vi "Add_Update_Values.vi"(0 "Filename":path, 1 "Value  Constant?":bool, 2 "Edit Raw data files?":bool, 3 "Filetype":string, 5 "New Chs In":string[](array[string])=[""], 7 "Edit Raw Data Header Info":bool, 9 "New Values In":string[][](array[string]), 11 "Selected Rows":i32[](array[numeric]), 12 "Edit all Rows?":bool, 13 "Raw DF in Orig Pos?":bool, 14 "Job Directory":path=path "/G4_2_HD/Users/paulhayden/Documents/Projects/Hong Roughness/XW data/XW_Corr.tpt") -> ()   [LabVIEW 2021]
panel:
  in  "Warn If files not found?":bool=TRUE
  out "Checking Raw data files":i32
  in  "stop":bool
  out "Currently editing":string
  out "Folder Containing Raw data Files":path
  out "size(s)":i32
  out "Files Processed":i32(slide) scale=0.0..522.0
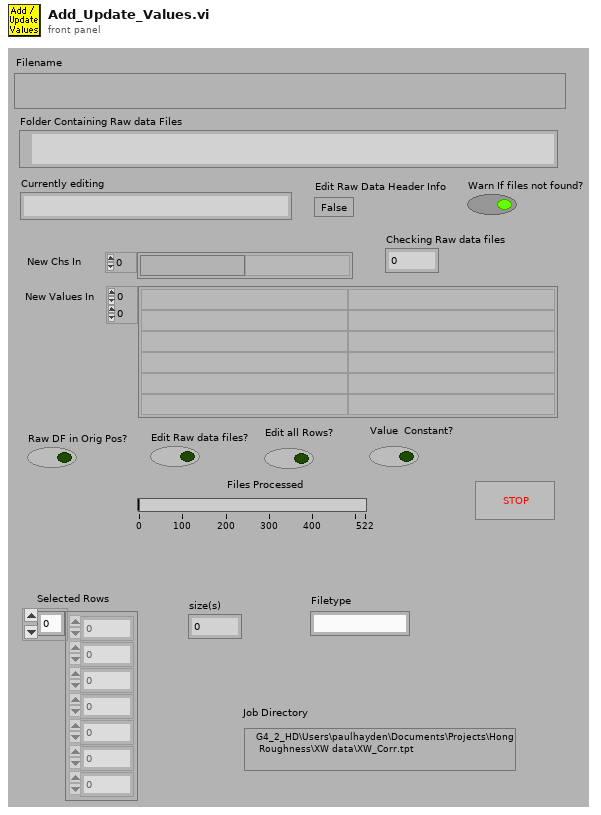
[diagram p1: front panel]
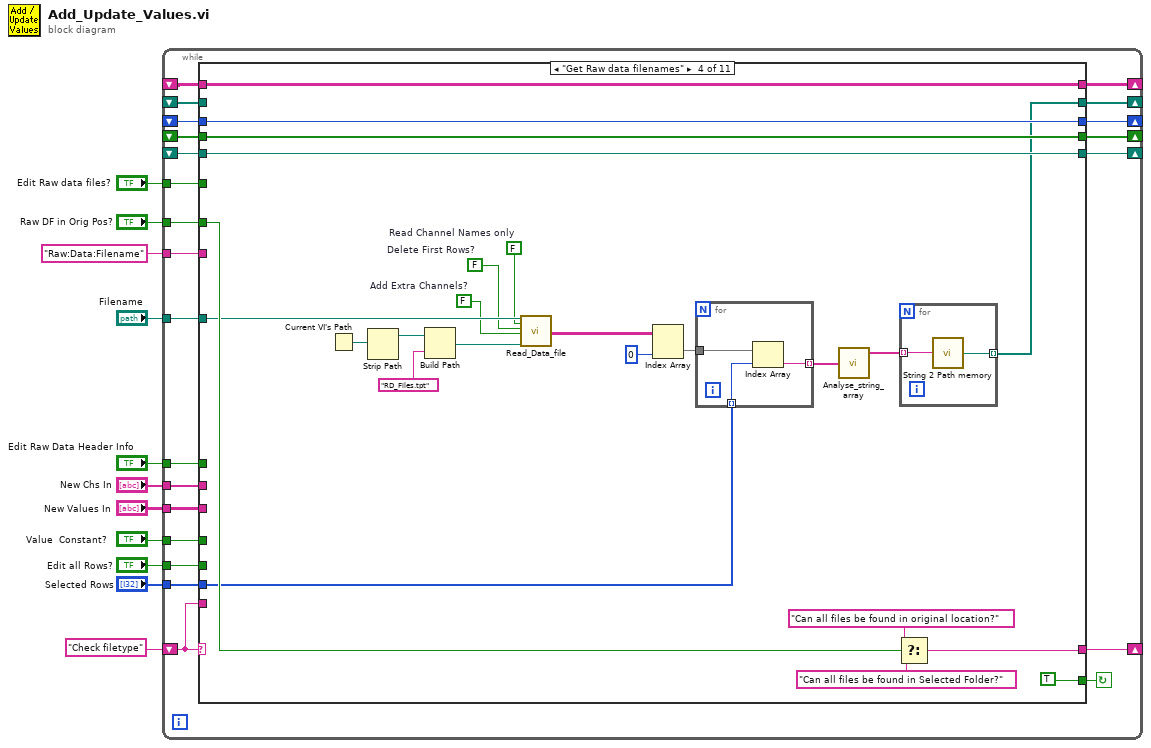
[diagram p0: block diagram]
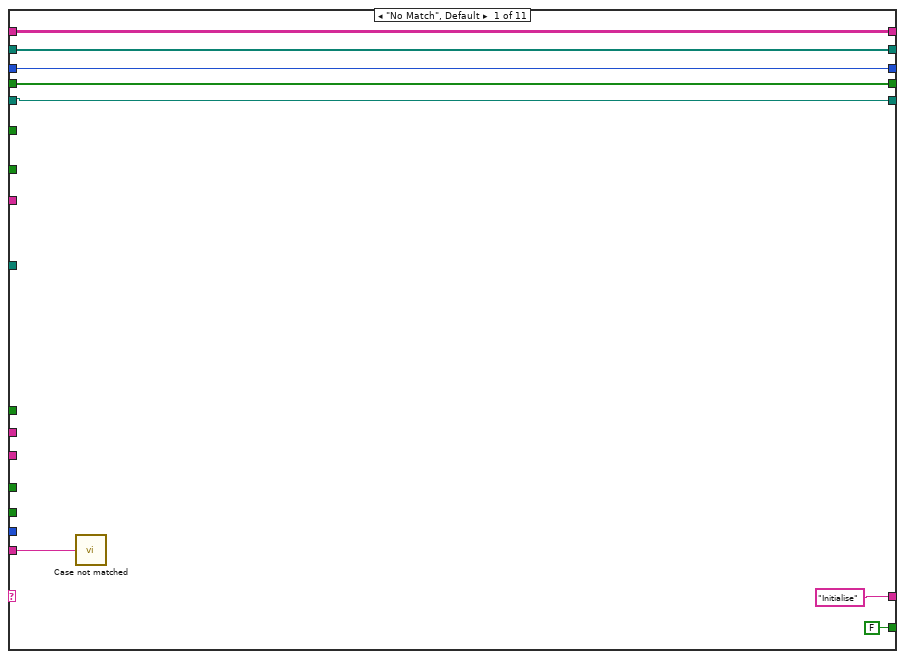
[diagram p2: hidden frame]
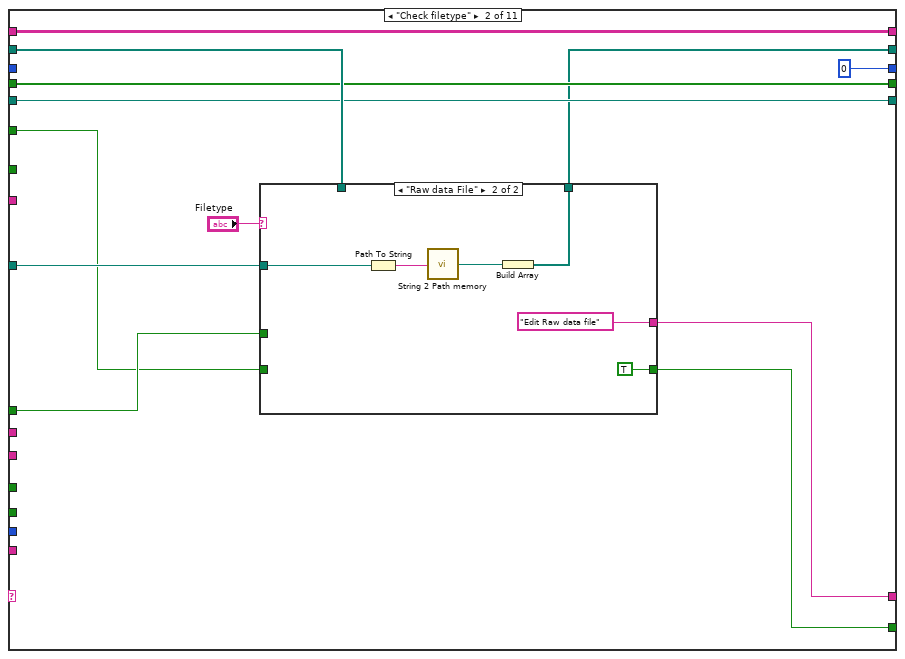
[diagram p3: hidden frame]
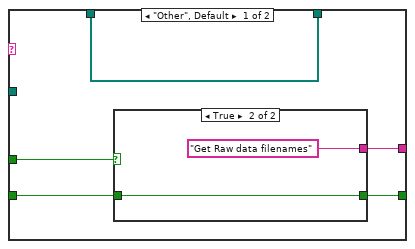
[diagram p4: hidden frame]
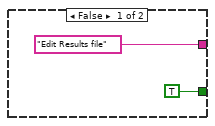
[diagram p5: hidden frame]
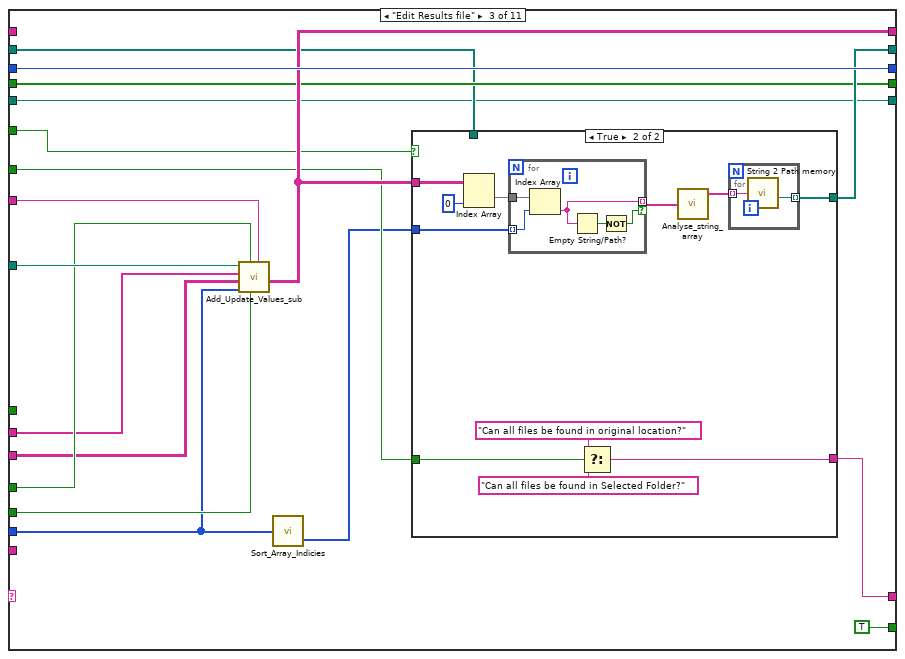
[diagram p6: hidden frame]
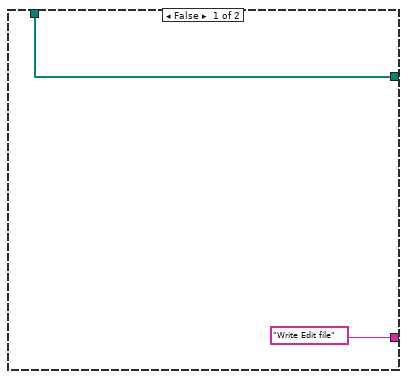
[diagram p7: hidden frame]
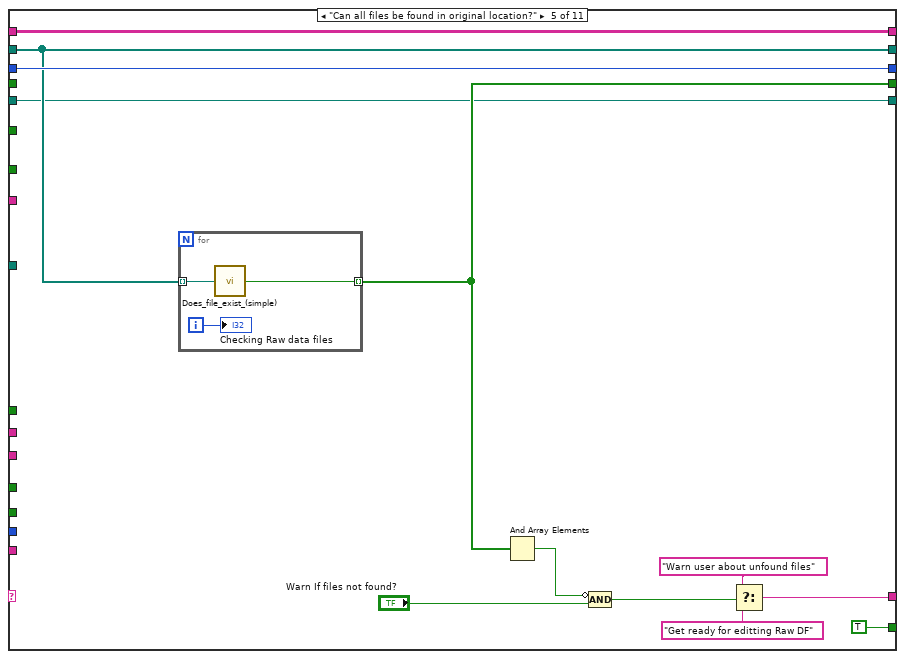
[diagram p8: hidden frame]
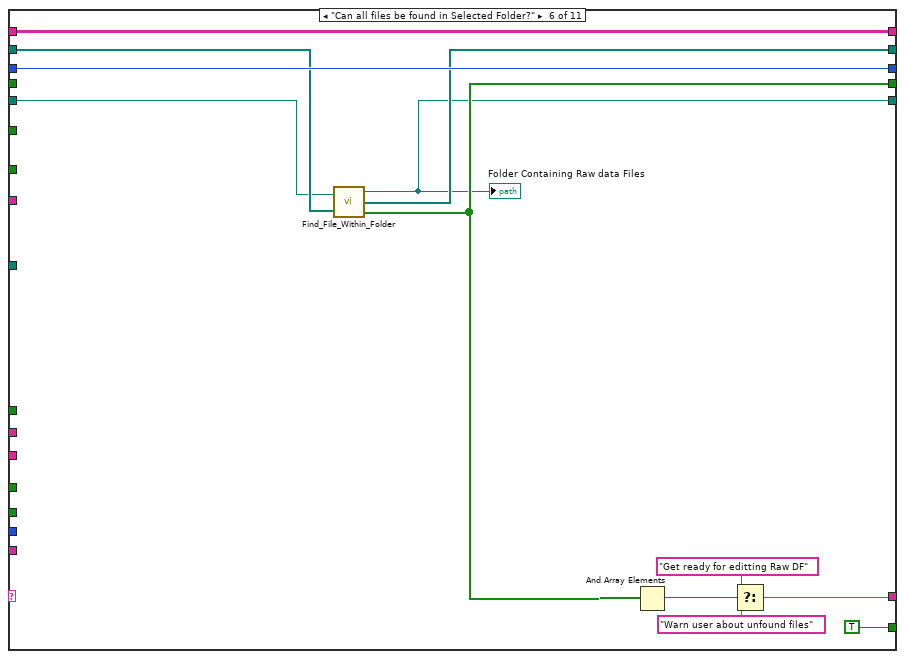
[diagram p9: hidden frame]
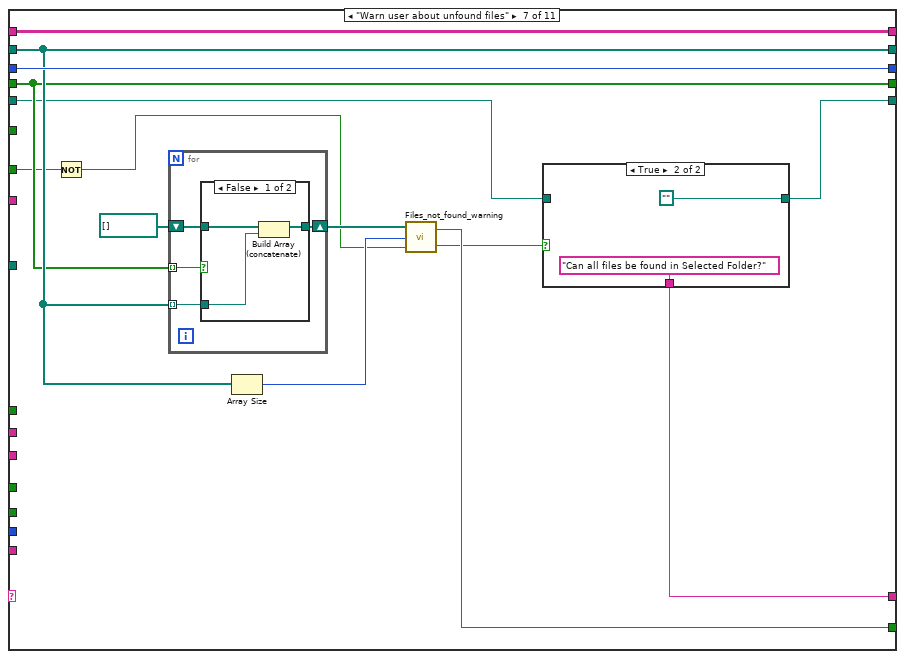
[diagram p10: hidden frame]
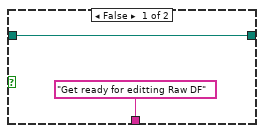
[diagram p11: hidden frame]
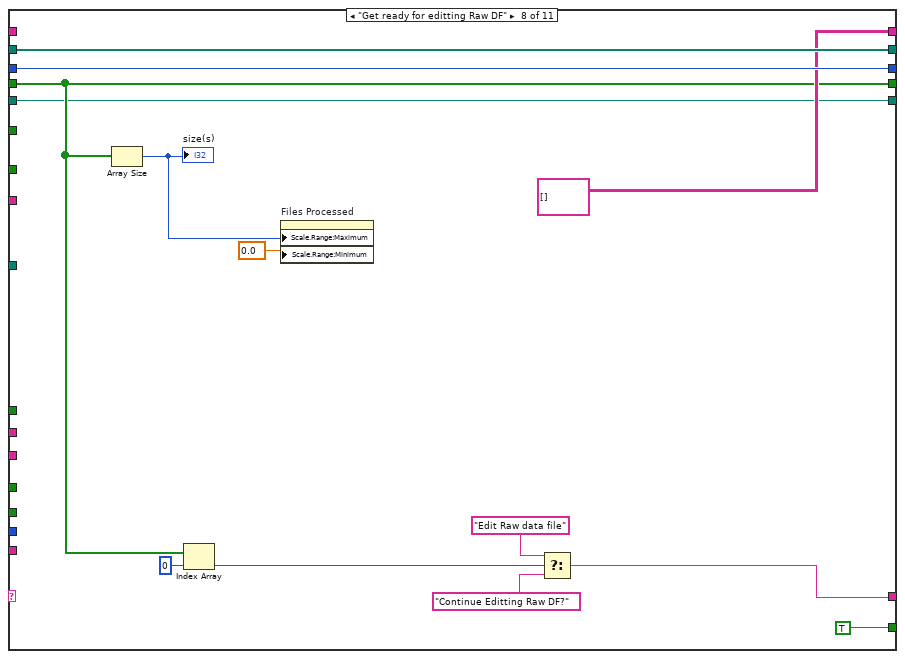
[diagram p13: hidden frame]
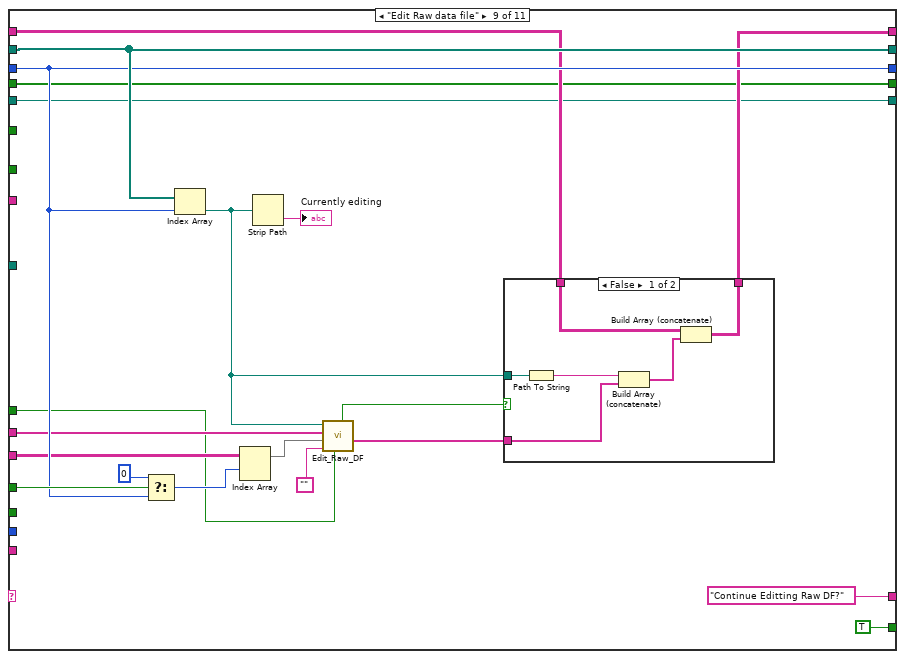
[diagram p14: hidden frame]
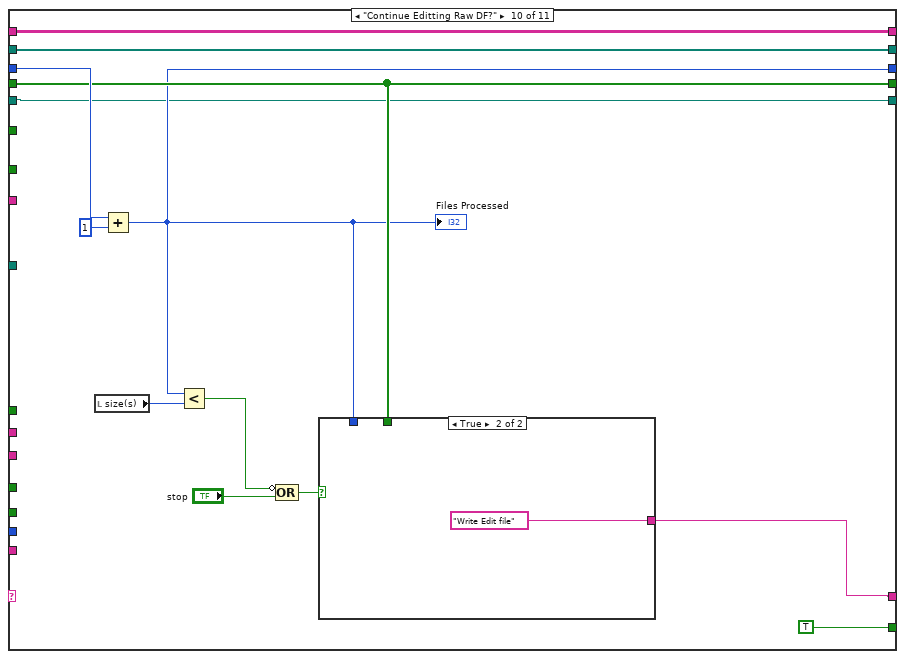
[diagram p16: hidden frame]
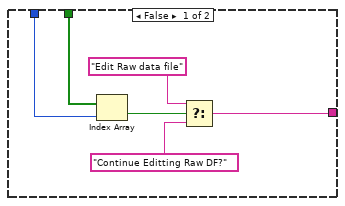
[diagram p17: hidden frame]
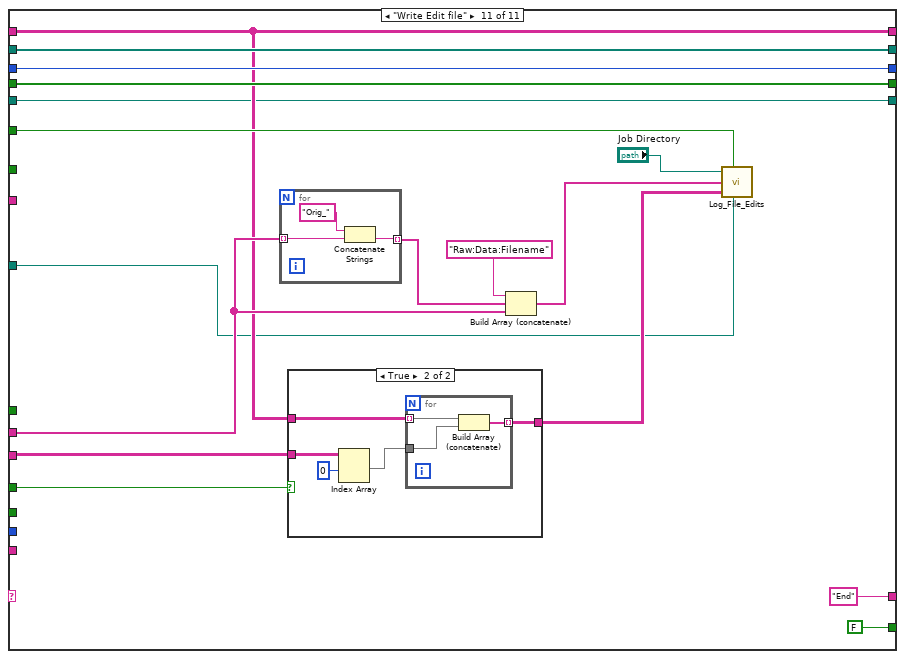
[diagram p18: hidden frame]
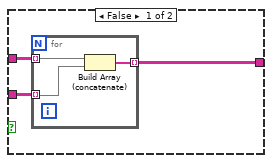
[diagram p19: hidden frame]
diagram:
  n1 = while {
    shift-left: "Check filetype" -> [w32]
    shift-right: [w33] -> _
    shift-right: [w30] -> _
    shift-left: _ -> [w29]
    tunnel: "Filename" -> [w31]
    shift-right: [w28] -> _
    shift-left: _ -> [w27]
    tunnel: "Value  Constant?" -> [w26]
    tunnel: "Edit Raw Data Header Info" -> [w25]
    shift-right: [w24] -> _
    shift-left: _ -> [w23]
    tunnel: "New Chs In" -> [w22]
    tunnel: "New Values In" -> [w21]
    tunnel: "Edit all Rows?" -> [w20]
    shift-right: [w19] -> _
    shift-left: _ -> [w18]
    tunnel: "Edit Raw data files?" -> [w17]
    tunnel: "Raw DF in Orig Pos?" -> [w16]
    shift-right: [w14] -> _
    shift-left: _ -> [w15]
    tunnel: "Selected Rows" -> [w13]
    tunnel: "Raw:Data:Filename" -> [w12]
    stop <- w34 continue-if-true
    n2 = case shown="\"Get Raw data filenames\"" w32 {
      tunnel: [FALSE w45 TRUE TRUE TRUE TRUE w171 TRUE TRUE TRUE FALSE] -> w34
      tunnel: ["Initialise" w52 w76 w128 w143 w154 w167 w194 "Continue Editting Raw DF?" ("t") w234 "End" ("t")] -> w33
      tunnel: w32 -> [w35 _ _ _ _ _ _ _ _ _ _]
      tunnel: w31 -> [_ w50 w85 w117 _ _ _ _ _ _ w252]
      tunnel: [w39 w43 w79 w111 w146 w160 w173 w200 w219 w240 w265] -> w30
      tunnel: w29 -> [w39 w53 w75 _ w146 w159 w173 w200 w219 w240 w265]
      tunnel: [w40 0 w87 w131 w148 w163 w177 w202 w218 w235 w263] -> w28
      tunnel: w27 -> [w40 _ w87 w131 w148 w163 w177 w202 w218 w239 w263]
      tunnel: w26 -> [_ _ w84 _ _ _ _ _ w222 _ w253]
      tunnel: w25 -> [_ w46 _ _ _ _ _ _ w204 _ _]
      tunnel: [w38 w49 w80 w123 w145 w161 w175 string[][] [] ("Edit Info") w209 w241 w256] -> w24
      tunnel: w23 -> [w38 w49 _ w123 w145 w161 w175 _ w210 w241 w256]
      tunnel: w22 -> [_ _ w83 _ _ _ _ _ w216 _ w258]
      tunnel: w21 -> [_ _ w82 _ _ _ _ _ w215 _ w255]
      tunnel: w20 -> [_ _ w81 _ _ _ _ _ _ _ _]
      tunnel: [w37 w48 w78 w129 w144 w155 w172 w198 w208 w236 w264] -> w19
      tunnel: w18 -> [w37 w48 w78 w129 _ _ w172 w198 w208 w236 w264]
      tunnel: w17 -> [_ w44 w77 _ _ _ _ _ _ _ w260]
      tunnel: w16 -> [_ _ w74 w127 _ _ w170 _ _ _ _]
      tunnel: w15 -> [w36 w47 w73 w126 w142 w153 w164 w190 w205 w230 w250]
      tunnel: [w36 w47 w73 w126 w142 w152 w165 w190 w205 w230 w250] -> w14
      tunnel: w13 -> [_ _ w71 w122 _ _ _ _ _ _ _]
      tunnel: w12 -> [_ _ w72 _ _ _ _ _ _ _ _]
      frame "No Match", Default {
        n3 = call "Case not matched.vi"("Case Name not Matched"=w35) -> ()
      }
      frame "Check filetype" {
        n4 = case shown="\"Raw data File\"" "Filetype" {
          tunnel: w50 -> [_ w67]
          tunnel: w53 -> [w55 _]
          tunnel: [w58 "Edit Raw data file"] -> w52
          tunnel: w46 -> [w59 _]
          tunnel: [w57 TRUE ("Edit Raw data files?")] -> w45
          tunnel: w44 -> [w56 _]
          tunnel: [w55 w64] -> w43
          frame "Other", Default {
            n5 = case shown="True" w59 {
              tunnel: ["Edit Results file" "Get Raw data filenames"] -> w58
              tunnel: [TRUE ("Edit Raw data files?") w62] -> w57
              tunnel: w56 -> [_ w62]
              frame False {
              }
              frame True {
              }
            }
          }
          frame "Raw data File" {
            n6 = Path To String(path=w67) -> (string=w66:string)
            n7 = call "String 2 Path memory.vi"("Input String"=w66) -> ("path"=w65:path)  [unwired: 1 in]
            n8 = Build Array(w65) -> (w64:path[])
          }
        }
      }
      frame "Edit Results file" {
        n9 = call "Add_Update_Values_sub.vi"("Raw data Filename column name"=w72, "Edit all Rows?"=w81, "Value  Constant?"=w84, "Selected Rows"=w71, "New Values In"=w82, "New Chs In"=w83, "Filename"=w85) -> ("Edit Info"=w80:string[][])  [unwired: 4 out]
        n10 = call "Sort_Array_Indicies.vi"("unsorted array"=w71) -> ("Sort Index"=w70:i32[])  [unwired: 1 out]
        n11 = case shown="True" w77 {
          tunnel: w80 -> [_ w100]
          tunnel: [w88 w90] -> w79
          tunnel: w74 -> [_ w98]
          tunnel: ["Write Edit file" w95] -> w76
          tunnel: w75 -> [w88 _]
          tunnel: w70 -> [_ w93]
          frame False {
          }
          frame True {
            n12 = Index Array(array=w100, index (col)=0 ("disabled index (col)")) -> (element=w94:string[])  [unwired: 1 in]
            n13 = for {
              tunnel: [w103] -> w92 mode=indexing if=w104
              tunnel: w94 -> [w107]
              tunnel: w93 -> [w106] mode=indexing
              n14 = Index Array(array=w107, index=w106) -> (element=w103:string)
              n15 = Empty String/Path?(string/path=w103) -> (empty?=w105:bool)
              n16 = Not(x=w105) -> (.not. x?=w104:bool)
            }
            n17 = Select(t="Can all files be found in original location?", s=w98, f="Can all files be found in Selected Folder?") -> (s? t:f=w95:string)
            n18 = call "Analyse_string_array.vi"("String array"=w92) -> ("Unique strings"=w91:string[])  [unwired: 1 in, 1 out]
            n19 = for {
              tunnel: [w102] -> w90 mode=indexing
              tunnel: w91 -> [w101] mode=indexing
              n20 = call "String 2 Path memory.vi"("Input String"=w101) -> ("path"=w102:path)  [unwired: 1 in]
            }
          }
        }
      }
      frame "Get Raw data filenames" {
        w110 = FALSE  # Delete First Rows?
        w114 = FALSE  # Add Extra Channels?
        w115 = FALSE  # Read Channel Names only
        n21 = Current VI's Path() -> (path=w120:path)
        n22 = Strip Path(path=w120) -> (stripped path=w119:path)  [unwired: 1 out]
        n23 = Build Path(base path=w119, name or relative path="RD_Files.tpt") -> (appended path=w116:path)
        n24 = call "Read_Data_file.vi"("Results file"=w117, "Read Channel Names only"=w115, "Delete First Rows?"=w110, "Add Extra Channels?"=w114, "Template File"=w116) -> ("Channel Values Out"=w113:string[][])  [unwired: 2 in, 12 out]
        n25 = Index Array(array=w113, index (col)=0 ("index (row)")) -> (element=w121:string[])  [unwired: 1 in]
        n26 = for {
          tunnel: w122 -> [w136] mode=indexing
          tunnel: w121 -> [w135]
          tunnel: [w134] -> w109 mode=indexing
          n27 = Index Array(array=w135, index=w136) -> (element=w134:string)
        }
        n28 = call "Analyse_string_array.vi"("String array"=w109) -> ("Unique strings"=w108:string[])  [unwired: 1 in, 1 out]
        n29 = Select(t="Can all files be found in original location?", s=w127, f="Can all files be found in Selected Folder?") -> (s? t:f=w128:string)
        n30 = for {
          tunnel: [w133] -> w111 mode=indexing
          tunnel: w108 -> [w132] mode=indexing
          n31 = call "String 2 Path memory.vi"("Input String"=w132) -> ("path"=w133:path)  [unwired: 1 in]
        }
      }
      frame "Can all files be found in original location?" {
        n32 = for {
          tunnel: w146 -> [w151] mode=indexing
          tunnel: [w150] -> w144 mode=indexing
          i -> [w149]
          n33 = call "Does_file_exist_(simple).vi"("Pathname"=w151) -> ("exists?"=w150:bool)
          "Checking Raw data files" <- w149
        }
        n34 = And Array Elements(Boolean array=w144) -> (logical AND=w141:bool)
        n35 = Compound Arithmetic op=AND(invert w141, "Warn If files not found?") -> (w139:bool)
        n36 = Select(t="Warn user about unfound files", s=w139, f="Get ready for editting Raw DF" ("t")) -> (s? t:f=w143:string)
      }
      frame "Can all files be found in Selected Folder?" {
        n37 = call "Find_File_Within_Folder.vi"("Folder to Search"=w153, "Files to find"=w159) -> ("Folder to Search Out"=w152:path, "New File Paths"=w160:path[], "Files Found?"=w155:bool[])
        "Folder Containing Raw data Files" <- w152
        n38 = And Array Elements(Boolean array=w155) -> (logical AND=w158:bool)
        n39 = Select(t="Get ready for editting Raw DF", s=w158, f="Warn user about unfound files") -> (s? t:f=w154:string)
      }
      frame "Warn user about unfound files" {
        n40 = Not(x=w170) -> (.not. x?=w169:bool)
        n41 = for {
          tunnel: w173 -> [w182] mode=indexing
          shift-right: [w185] -> w174
          shift-left: path[] [] -> [w184]
          tunnel: w172 -> [w183] mode=indexing
          n42 = case shown="False" w183 {
            tunnel: w184 -> [w188 w189]
            tunnel: [w186 w189] -> w185
            tunnel: w182 -> [w187 _]
            frame False {
              n43 = Build Array (concatenate)(w188, w187) -> (w186:path[])
            }
            frame True {
            }
          }
        }
        n44 = Array Size(array=w173) -> (size(s)=w176:i32)
        n45 = call "Files_not_found_warning.vi"("Use Selected Folder?"=w169, "Total number of data files"=w176, "Unfound Files"=w174) -> ("Edit Selected Folder Out"=w168:bool, "Edit Files?"=w171:bool)
        n46 = case shown="True" w168 {
          tunnel: ["Get ready for editting Raw DF" ("t") "Can all files be found in Selected Folder?" ("t")] -> w167
          tunnel: [w178 path ""] -> w165
          tunnel: w164 -> [w178 _]
          frame False {
          }
          frame True {
          }
        }
      }
      frame "Get ready for editting Raw DF" {
        n47 = Array Size(array=w198) -> (size(s)=w191:i32)
        "size(s)" <- w191
        n48 = Index Array(array=w198, index=0) -> (element=w196:bool)
        n49 = property on="Files Processed" class="Slide (strict)"("Scale.Range:Maximum"=w191, "Scale.Range:Minimum"=0.0 ("Scale.Range:Maximum")) -> ()  [unwired: 2 in, 2 out]
        n50 = Select(t="Edit Raw data file", s=w196, f="Continue Editting Raw DF?") -> (s? t:f=w194:string)
      }
      frame "Edit Raw data file" {
        n51 = Select(t=0, s=w222, f=w218) -> (s? t:f=w220:i32)
        n52 = Index Array(array=w219, index=w218) -> (element=w207:path)
        n53 = Index Array(array=w215, index (row)=w220) -> (element=w214:string[])  [unwired: 1 in]
        n54 = Strip Path(path=w207) -> (name=→"Currently editing":string)  [unwired: 1 out]
        n55 = call "Edit_Raw_DF.vi"("Edit Raw Data Header Info"=w204, "New Analysis Info Cluster Setup"="", "New Values In"=w214, "New Chs In"=w216, "Data filename"=w207) -> ("Original values"=w212:string[], "File Not Changed?"=w211:bool)  [unwired: 1 in, 2 out]
        n56 = case shown="False" w211 {
          tunnel: w207 -> [w228 _]
          tunnel: w212 -> [w226 _]
          tunnel: w210 -> [w224 w229]
          tunnel: [w223 w229] -> w209
          frame False {
            n57 = Path To String(path=w228) -> (string=w227:string)
            n58 = Build Array (concatenate)(w227, w226) -> (w225:string[])
            n59 = Build Array (concatenate)(w224, w225) -> (w223:string[][])
          }
          frame True {
          }
        }
      }
      frame "Continue Editting Raw DF?" {
        n60 = local read "size(s)"() -> (w237:i32)
        n61 = Add(x=w239, y=1) -> (x+y=w235:i32)
        "Files Processed" <- w235
        n62 = Less?(x=w235, y=w237) -> (x < y?=w232:bool)
        n63 = Compound Arithmetic op=OR(invert w232, "stop") -> (w231:bool)
        n64 = case shown="True" w231 {
          tunnel: w236 -> [w247 _]
          tunnel: w235 -> [w246 _]
          tunnel: [w244 "Write Edit file" ("t")] -> w234
          frame False {
            n65 = Index Array(array=w247, index=w246) -> (element=w248:bool)
            n66 = Select(t="Edit Raw data file", s=w248, f="Continue Editting Raw DF?") -> (s? t:f=w244:string)
          }
          frame True {
          }
        }
      }
      frame "Write Edit file" {
        n67 = for {
          tunnel: w258 -> [w283] mode=indexing
          tunnel: [w281] -> w259 mode=indexing
          n68 = Concatenate Strings("Orig_" ("string"), w283) -> (w281:string)
        }
        n69 = case shown="True" w253 {
          tunnel: w256 -> [w269 w277]
          tunnel: w255 -> [w268 w275]
          tunnel: [w267 w276] -> w254
          frame False {
            n70 = for {
              tunnel: w269 -> [w272] mode=indexing
              tunnel: w268 -> [w271] mode=indexing
              tunnel: [w270] -> w267 mode=indexing
              n71 = Build Array (concatenate)(w272, w271) -> (w270:string[])
            }
          }
          frame True {
            n72 = Index Array(array=w275, index (row)=0) -> (element=w273:string[])  [unwired: 1 in]
            n73 = for {
              tunnel: w277 -> [w280] mode=indexing
              tunnel: [w279] -> w276 mode=indexing
              tunnel: w273 -> [w278]
              n74 = Build Array (concatenate)(w280, w278) -> (w279:string[])
            }
          }
        }
        n75 = Build Array (concatenate)("Raw:Data:Filename", w259, w258) -> (w257:string[])
        n76 = call "Log_File_Edits.vi"("Job Directory"="Job Directory", "File Editted?"=w260, "Channels to Edit"=w257, "Data"=w254, "Results file name"=w252) -> ()  [unwired: 2 out]
      }
    }
  }
